vi "GenerateDGMLExternalFolderString.vi"(5 "Apply? (T)":bool=TRUE, 7 "ILabVIEWItem in":refnum<class "ILabVIEWItem.lvclass">, 8 "Links in":T1, 9 "Nodes in":T1, 10 "Path in":string="Z:\\OtherFiles", 11 "CGrapherDGML in":refnum<class "CGrapherDGML.lvclass">) -> (0 "Links":T1, 1 "Nodes":T1, 3 "CGrapherDGML":refnum<class "CGrapherDGML.lvclass">)   [LabVIEW 2020, in "DefaultExtensions.lvlib" / "CGrapherDGML.lvclass"]
uses:
  CGrapherDGML.lvclass
  LabVIEWObjectInterfaces/ILabVIEWItem/ILabVIEWItem.lvclass
  LabVIEWItem/CLabVIEWItem/ConnectionSet.ctl
  CGrapherDGML.lvclass/CGrapherDGML.ctl
  ecf4d353-cf80-4459-a486-8bebc84a9ab0.vi
  LabVIEWItem/CLabVIEWItem/CLabVIEWItem.lvclass
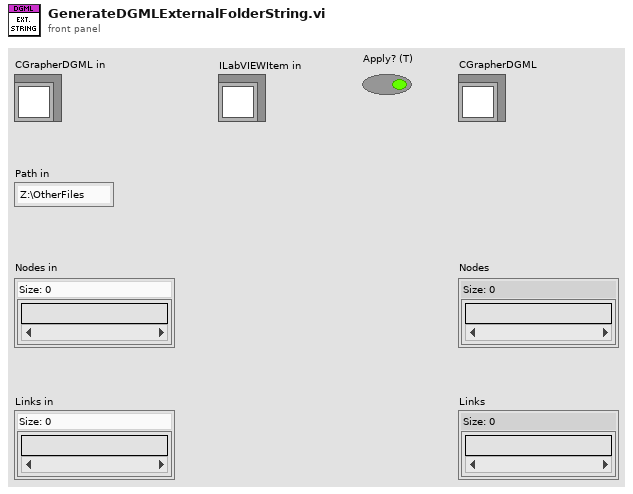
[diagram p1: front panel]
types:
  T1 = typedef "LabVIEWItem.lvlib/CLabVIEWItem.lvclass/ConnectionSet.ctl" = set{string}
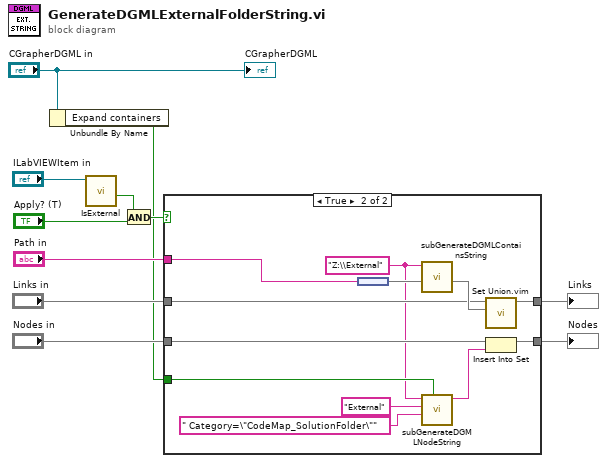
[diagram p0: block diagram]
diagram:
  n1 = Unbundle By Name("CGrapherDGML in") -> ("Expand containers"=w1:bool)
  n2 = call-dynamic "IsExternal.vi"("ILabVIEWItem in"="ILabVIEWItem in") -> ("Is external?"=w5:bool)  [unwired: 8 in, 2 out]
  n3 = And(x=w5, y="Apply? (T)") -> (x .and. y?=w3:bool)
  n4 = case shown="True" w3 {
    tunnel: [w13 w20] -> w11
    tunnel: "Links in" -> [w13 w19]
    tunnel: "Nodes in" -> [w12 w18]
    tunnel: [w12 w17] -> w8
    tunnel: w1 -> [_ w16]
    tunnel: "Path in" -> [_ w15]
    frame False {
    }
    frame True {
      w14 = "Z:\\External" ("format string")
      n5 = node(w15) -> (w25:set{string})
      n6 = call "subGenerateDGMLContainsString.vi"("Contained"=w25, "Source"=w14) -> ("Links"=w24:T1)  [unwired: 9 in]
      n7 = call "subGenerateDGMLNodeString.vi"("Expand?"=w16, "Code schema"=" Category=\"CodeMap_SolutionFolder\"" ("format string"), "Label"="External" ("format string"), "Id"=w14) -> ("Node string"=w22:string)  [unwired: 7 in]
      n8 = call "Set Union.vim"("set 2"=w24, "set 1"=w19) -> ("union"=w20:T1)  [unwired: 9 in]
      n9 = Insert Into Set(10:w22, 11:w18) -> (3:w17:T1)  [unwired: 1 out]
    }
  }
  "Links" <- w11
  "Nodes" <- w8
  "CGrapherDGML" <- "CGrapherDGML in"
